vi "I_Read_position(old).vi"(2 "Axis":enum16{"X", "Y", "Z"}(ring), 3 "Motor GPIB":u8=6 max=100) -> (0 "Error?":bool, 1 "Position":i32)   [LabVIEW 2010]
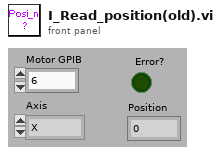
[diagram p1: front panel]
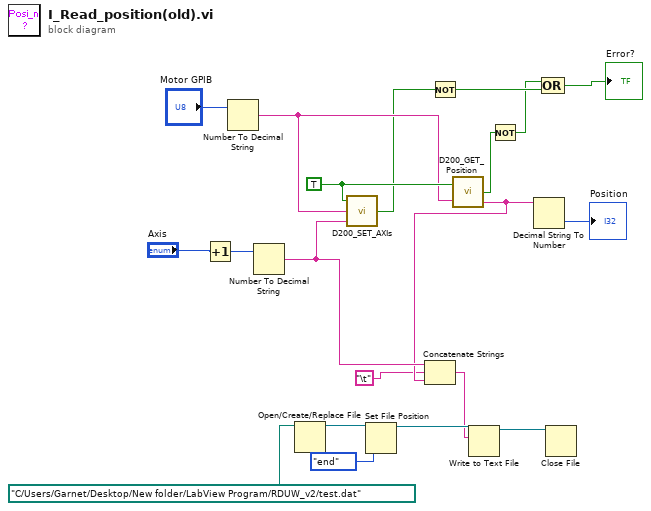
[diagram p0: block diagram]
diagram:
  w20 = TRUE ("Permission")
  n1 = Increment(x="Axis") -> (x+1=w17:enum16{"X", "Y", "Z"})
  n2 = Number To Decimal String(number="Motor GPIB") -> (decimal integer string=w15:string)  [unwired: 1 in]
  n3 = Number To Decimal String(number=w17) -> (decimal integer string=w5:string)  [unwired: 1 in]
  n4 = Open/Create/Replace File(file path (use dialog)=path "C:/Users/Garnet/Desktop/New folder/LabView Program/RDUW_v2/test.dat") -> (refnum out=w9:refnum<file>)  [unwired: 5 in, 2 out]
  n5 = call "D200_SET_AXIs.vi"("Axis No"=w5, "GPIB Addr"=w15, "Permission"=w20) -> ("Finish Write"=w14:bool)
  n6 = Set File Position(refnum=w9, from (0:start)=enum16{"start", "end", "current"}."end") -> (refnum out=w7:refnum<file>)  [unwired: 2 in, 1 out]
  n7 = Not(x=w14) -> (.not. x?=w13:bool)
  n8 = call "D200_GET_Position.vi"("Permission"=w20, "GPIB Addr"=w15) -> ("Finish Read"=w12:bool, "Current position"=w4:string)  [unwired: 1 out]
  n9 = Concatenate Strings(w5, "\t", w4) -> (w6:string)
  n10 = Write to Text File(file (use dialog)=w7, text=w6) -> (refnum out=w3:refnum<file>)  [unwired: 2 in, 2 out]
  n11 = Not(x=w12) -> (.not. x?=w11:bool)
  n12 = Decimal String To Number(string=w4) -> (number=→"Position":i32)  [unwired: 2 in, 1 out]
  n13 = Compound Arithmetic op=OR(w11, w13) -> (→"Error?":bool)
  n14 = Close File(refnum=w3) -> ()  [unwired: 1 in, 2 out]
